vi "Routing_change.vi"(5 "Part":T2, 6 "Routing?Pokayoke":bool, 7 "Line":T2, 8 "error in (no error)":errorcluster, 11 "Ref In":T1) -> (0 "error out":errorcluster)   [LabVIEW 2020]
uses:
  Controls/Roting.ctl
  <menus>/Controls/Devaseelan Style/ONOFF Small.ctl
  <vilib>/addons/database/Connection.llb/Conn ObjectReference.ctl
  <vilib>/addons/database/Connection.llb/Conn Execute.vi
  <vilib>/addons/database/Recordset.llb/Rec Destroy - Connection.vi
  <vilib>/addons/database/NI_Database_API.lvlib
panel:
  out "spreadsheet string 2":string
  out "spreadsheet string":string
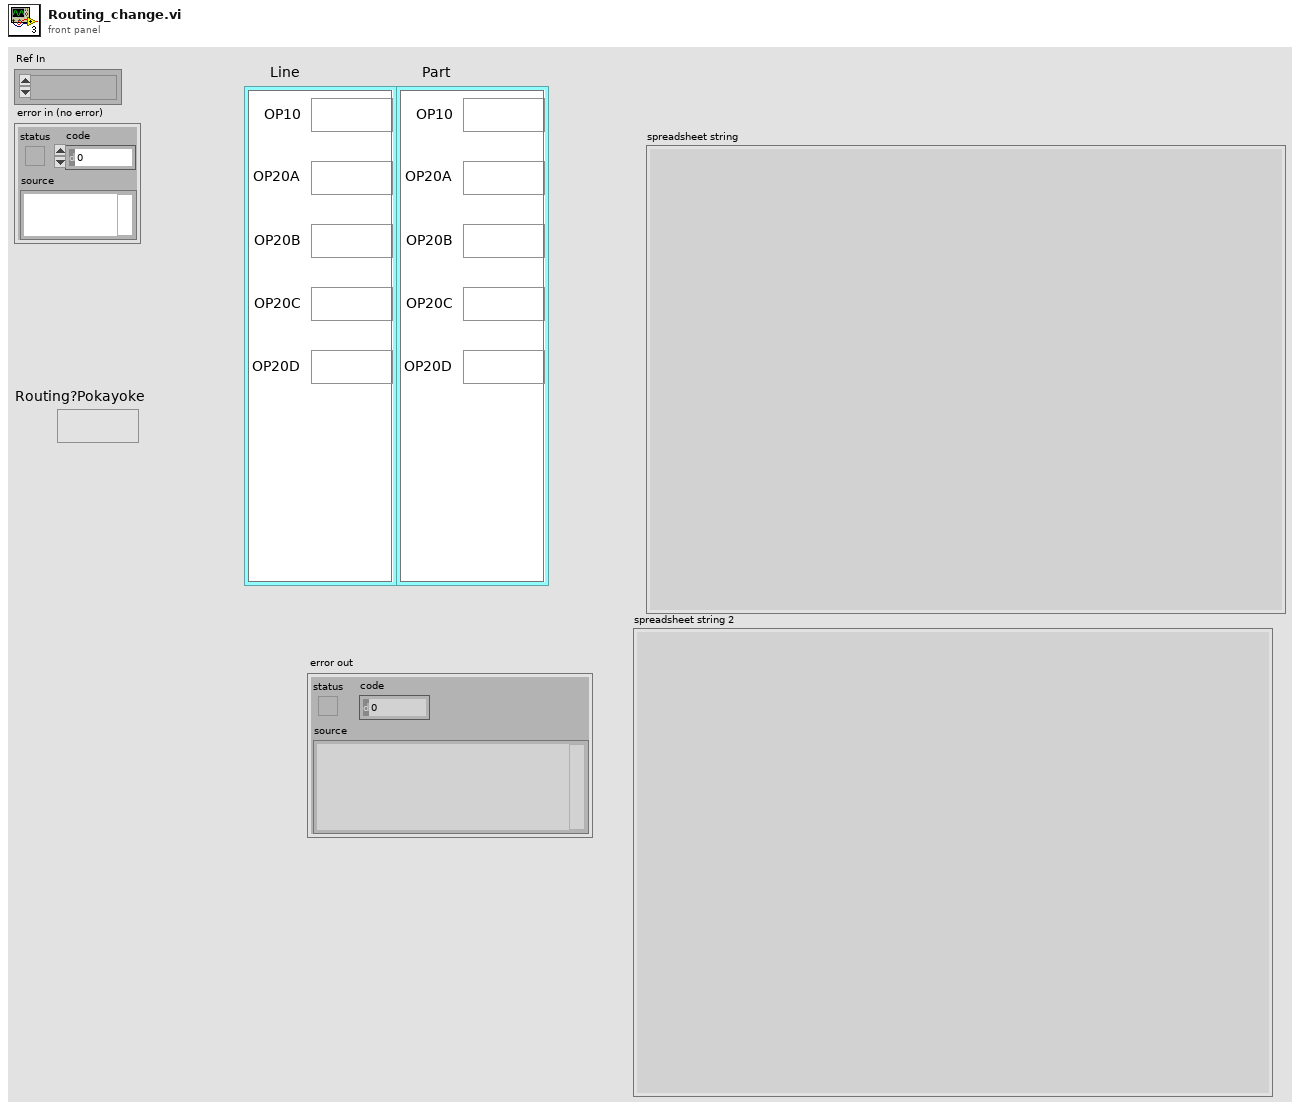
[diagram p1: front panel]
types:
  T1 = typedef "NI_Database_API.lvlib/Conn ObjectReference.ctl" = refnum<k1>
  T2 = typedef "Roting.ctl" = cluster{"OP10":T3, "OP20A":T3, "OP20B":T3, "OP20C":T3, "OP20D":T3}
  T3 = typedef "ONOFF Small.ctl" = bool
  T4 = typedef "NI_Database_API.lvlib/Rec ObjectReference.ctl" = refnum<k1>
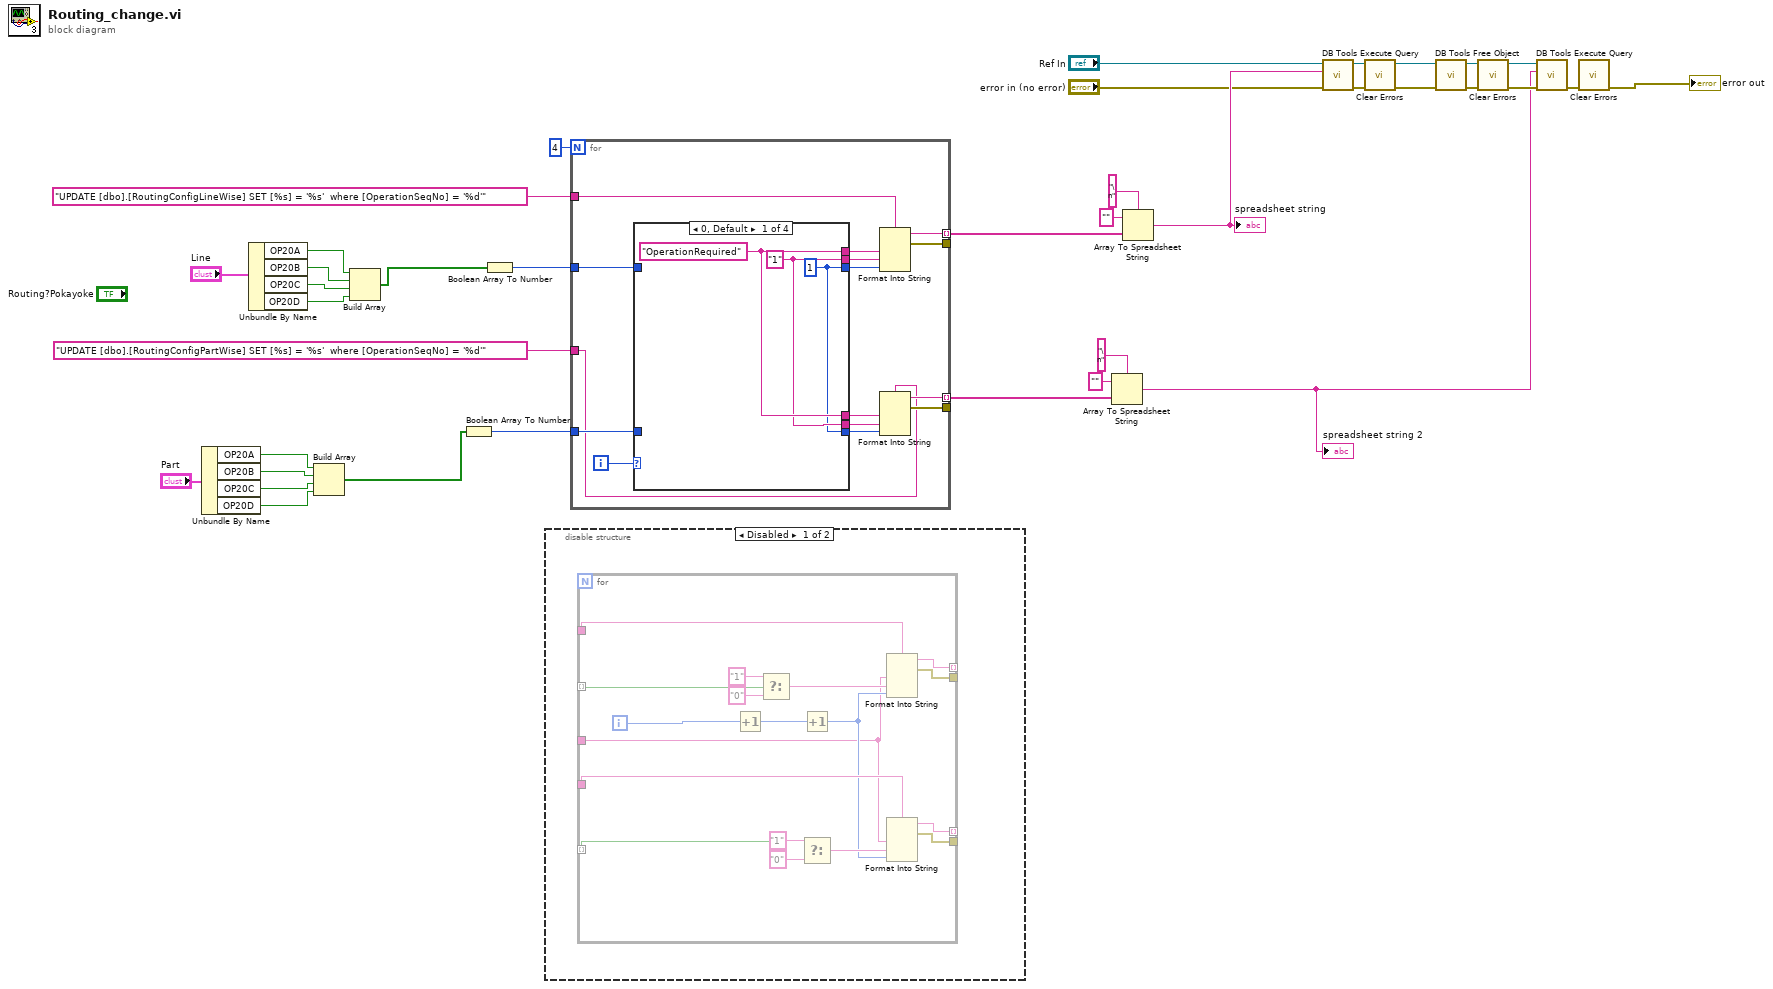
[diagram p0: block diagram]
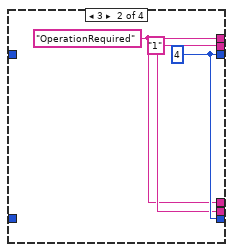
[diagram p3: hidden frame]
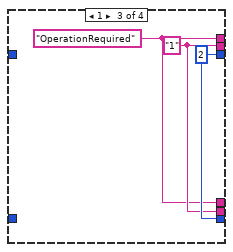
[diagram p4: hidden frame]
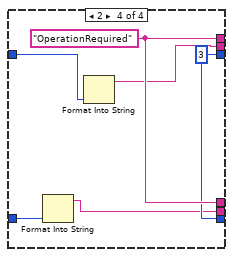
[diagram p5: hidden frame]
diagram:
  n1 = Unbundle By Name("Part") -> ("OP20A"=w11:T3, "OP20B"=w10:T3, "OP20C"=w9:T3, "OP20D"=w8:T3)
  n2 = Unbundle By Name("Line") -> ("OP20A"=w5:T3, "OP20B"=w4:T3, "OP20C"=w3:T3, "OP20D"=w2:T3)
  n3 = Build Array(w11, w10, w9, w8) -> (w7:T3[])
  n4 = Build Array(w5, w4, w3, w2) -> (w1:T3[])
  n5 = Boolean Array To Number(Boolean array=w7) -> (number=w15:u32)
  n6 = Boolean Array To Number(Boolean array=w1) -> (number=w14:u32)
  n7 = disable-structure shown="Disabled" {
    frame Disabled {
      n8 = for {
        tunnel: _ -> [w53] mode=indexing
        tunnel: _ -> [w50]
        tunnel: [w47] -> _
        tunnel: [w46] -> _ mode=indexing
        tunnel: _ -> [w42] mode=indexing
        tunnel: _ -> [w45]
        tunnel: [w39] -> _
        tunnel: [w38] -> _ mode=indexing
        tunnel: _ -> [w37]
        i -> [w36]
        n9 = Increment(x=w36) -> (x+1=w48:i32)
        n10 = Select(t="1", s=w53, f="0" ("SQL query")) -> (s? t:f=w49:string)
        n11 = Increment(x=w48) -> (x+1=w40:i32)
        n12 = Select(t="1", s=w42, f="0" ("SQL query")) -> (s? t:f=w41:string)
        n13 = Format Into String(format string=w50, w37, w49, w40) -> (resulting string=w46:string, error out=w47:errorcluster)  [unwired: 2 in]
        n14 = Format Into String(format string=w45, w37, w41, w40) -> (resulting string=w38:string, error out=w39:errorcluster)  [unwired: 2 in]
      }
    }
    frame Enabled {
    }
  }
  n15 = for {
    N: 4 -> [_]
    tunnel: "UPDATE [dbo].[RoutingConfigLineWise] SET [%s] = '%s'  where [OperationSeqNo] = '%d'" ("SQL query") -> [w68]
    tunnel: [w67] -> _
    tunnel: [w66] -> w34 mode=indexing
    tunnel: "UPDATE [dbo].[RoutingConfigPartWise] SET [%s] = '%s'  where [OperationSeqNo] = '%d'" ("SQL query") -> [w54]
    tunnel: [w65] -> _
    tunnel: [w64] -> w28 mode=indexing
    tunnel: w15 -> [w59]
    tunnel: w14 -> [w58]
    i -> [w63]
    n16 = case shown="0, Default" w63 {
      tunnel: [w69 w74 w77 w81] -> w62
      tunnel: [w71 w72 w75 w83] -> w61
      tunnel: [w70 w73 w76 w80] -> w60
      tunnel: w59 -> [_ _ _ w79]
      tunnel: [w69 w74 w77 w81] -> w57
      tunnel: w58 -> [_ _ _ w82]
      tunnel: [w71 w72 w75 w83] -> w56
      tunnel: [w70 w73 w76 w78] -> w55
      frame 0, Default {
        w69 = u32 1
        w71 = "OperationRequired"
        w70 = "1"
      }
      frame 3 {
        w74 = u32 4
        w72 = "OperationRequired"
        w73 = "1"
      }
      frame 1 {
        w77 = u32 2
        w75 = "OperationRequired"
        w76 = "1"
      }
      frame 2 {
        w81 = u32 3
        w83 = "OperationRequired"
        n17 = Format Into String(w79) -> (resulting string=w78:string)  [unwired: 3 in, 1 out]
        n18 = Format Into String(w82) -> (resulting string=w80:string)  [unwired: 3 in, 1 out]
      }
    }
    n19 = Format Into String(format string=w68, w61, w60, w57) -> (resulting string=w66:string, error out=w67:errorcluster)  [unwired: 2 in]
    n20 = Format Into String(format string=w54, w56, w55, w62) -> (resulting string=w64:string, error out=w65:errorcluster)  [unwired: 2 in]
  }
  n21 = Array To Spreadsheet String(delimiter (Tab)="\n", array=w28, 3:"" ("format string")) -> (spreadsheet string=w18:string)
  "spreadsheet string 2" <- w18
  n22 = Array To Spreadsheet String(delimiter (Tab)="\n", array=w34, 3:"" ("format string")) -> (spreadsheet string=w27:string)
  "spreadsheet string" <- w27
  n23 = call-poly <vilib>:"DB Tools Execute Query.vi"("error in (no error)"="error in (no error)", "SQL query"=w27, "connection reference"="Ref In") -> ("error out"=w22:errorcluster, "recordset reference"=w24:T4)  [unwired: 5 in]
  n24 = call <vilib>:"Clear Errors.vi"("error in (no error)"=w22) -> ("error out"=w21:errorcluster)  [unwired: 5 in, 1 out]
  n25 = call-poly <vilib>:"DB Tools Free Object.vi"("error in (no error)"=w21, "recordset reference"=w24) -> ("error out"=w20:errorcluster, "connection reference"=w23:T1)  [unwired: 8 in]
  n26 = call <vilib>:"Clear Errors.vi"("error in (no error)"=w20) -> ("error out"=w19:errorcluster)  [unwired: 5 in, 1 out]
  n27 = call-poly <vilib>:"DB Tools Execute Query.vi"("error in (no error)"=w19, "SQL query"=w18, "connection reference"=w23) -> ("error out"=w17:errorcluster)  [unwired: 5 in, 1 out]
  n28 = call <vilib>:"Clear Errors.vi"("error in (no error)"=w17) -> ("error out"=→"error out":errorcluster)  [unwired: 5 in, 1 out]
